vi "Detect_Hart_485_Ports.vi"(8 "error in (no error)":errorcluster) -> (0 "error out":errorcluster, 1 "total # ports found":i32, 2 "485 Ports":refnum<visa-resource-name>[](array[refnum]), 3 "HART ports":refnum<visa-resource-name>[](array[refnum]), 4 "# 485 ports found":i32, 5 "# HART ports found":i32)   [LabVIEW 2016]
uses:
  <vilib>/Instr/_visa.llb/VISA Find Search Mode.ctl
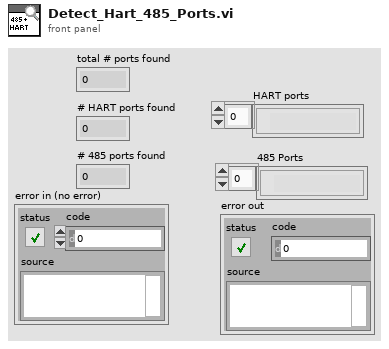
[diagram p1: front panel]
types:
  T1 = typedef "VISA Find Search Mode.ctl" = u32
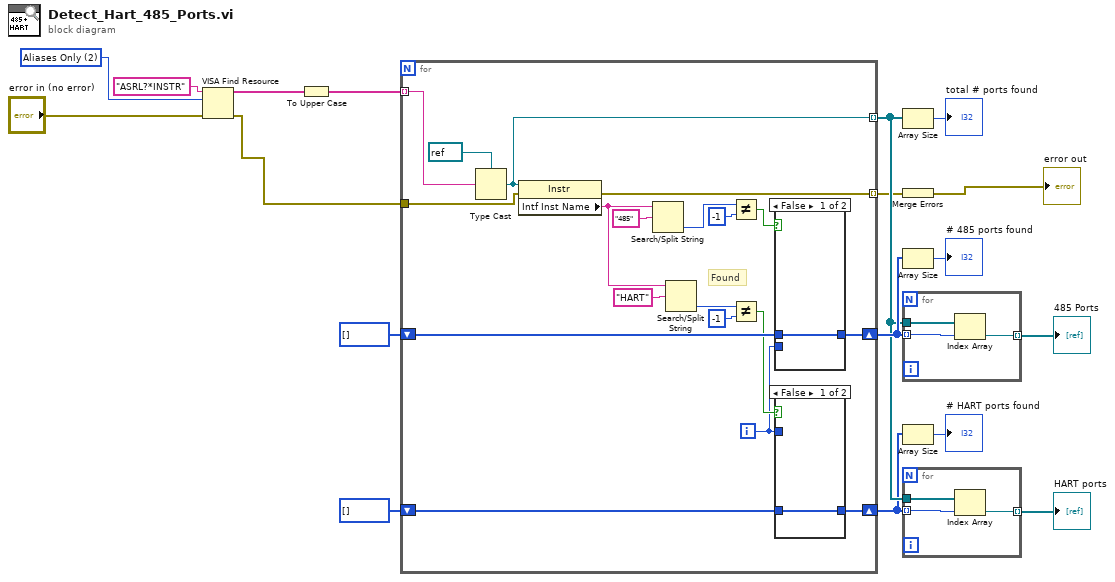
[diagram p0: block diagram]
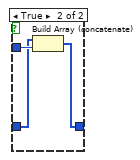
[diagram p2: hidden frame]
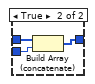
[diagram p3: hidden frame]
diagram:
  w6 = T1 2 items=["Canonical Names Only"=0, "Aliases Only"=2, "Include Matching Aliases"=3, "Include All Aliases"=4] ("Search Mode")
  n1 = VISA Find Resource(8:"error in (no error)", 10:w6, 11:"ASRL?*INSTR" ("expression (\"?*\")")) -> (0:w2:errorcluster, 3:w17:string[])  [unwired: 1 out]
  n2 = To Upper Case(1:w17) -> (0:w18:string[])
  n3 = for {
    tunnel: w18 -> [w37] mode=indexing
    shift-right: [w31] -> w12
    shift-left: i32[] [] -> [w30]
    shift-right: [w23] -> w7
    shift-left: i32[] [] -> [w22]
    tunnel: [w21] -> w10 mode=indexing
    tunnel: [w20] -> w3 mode=indexing
    tunnel: w2 -> [w19]
    i -> [w24]
    # "Found"
    n4 = Type Cast(type=refnum<visa-resource-name> refnum ("reference"), x=w37) -> (*(type *) &x=w21:refnum<visa-resource-name>)
    n5 = property class="Instr"(reference=w21, error in=w19) -> (error out=w20:errorcluster, "Intf Inst Name"=w29:string)  [unwired: 1 out]
    n6 = Search/Split String(string=w29, search string/char (-)="485") -> (offset of match=w35:i32)  [unwired: 1 in, 2 out]
    n7 = Search/Split String(string=w29, search string/char (-)="HART") -> (offset of match=w26:i32)  [unwired: 1 in, 2 out]
    n8 = Not Equal?(x=w35, y=-1) -> (x != y?=w32:bool)
    n9 = Not Equal?(x=w26, y=-1) -> (x != y?=w25:bool)
    n10 = case shown="False" w32 {
      tunnel: [w42 w45] -> w31
      tunnel: w24 -> [_ w44]
      tunnel: w30 -> [w42 w43]
      frame False {
      }
      frame True {
        n11 = Build Array (concatenate)(w43, w44) -> (w45:i32[])
      }
    }
    n12 = case shown="False" w25 {
      tunnel: [w38 w41] -> w23
      tunnel: w24 -> [_ w40]
      tunnel: w22 -> [w38 w39]
      frame False {
      }
      frame True {
        n13 = Build Array (concatenate)(w39, w40) -> (w41:i32[])
      }
    }
  }
  n14 = Array Size(array=w10) -> (size(s)=→"total # ports found":i32)
  n15 = Merge Errors(w3) -> (→"error out":errorcluster)
  n16 = Array Size(array=w12) -> (size(s)=→"# 485 ports found":i32)
  n17 = for {
    tunnel: w12 -> [w48] mode=indexing
    tunnel: w10 -> [w47]
    tunnel: [w46] -> w14 mode=indexing
    n18 = Index Array(array=w47, index=w48) -> (element=w46:refnum<visa-resource-name>)
  }
  "485 Ports" <- w14
  n19 = Array Size(array=w7) -> (size(s)=→"# HART ports found":i32)
  n20 = for {
    tunnel: w7 -> [w51] mode=indexing
    tunnel: [w50] -> w13 mode=indexing
    tunnel: w10 -> [w49]
    n21 = Index Array(array=w49, index=w51) -> (element=w50:refnum<visa-resource-name>)
  }
  "HART ports" <- w13
